vi "Calc Dev (DAQ Rack).vi"(0 "Verify Table IN":string[][](array[string]), 1 "Units":T2, 2 "Rack Version":T1, 5 "Dev Table 1 Ref":refnum<vi>) -> (14 "Verify Table OUT":string[][](array[string]))   [LabVIEW 2019]
uses:
  Type Defs/Units Type Def (DAQ Rack).ctl
  Type Defs/Rack Version Type Def.ctl
  <vilib>/Utility/miscctls.llb/LVRowAndColumnTypeDef.ctl
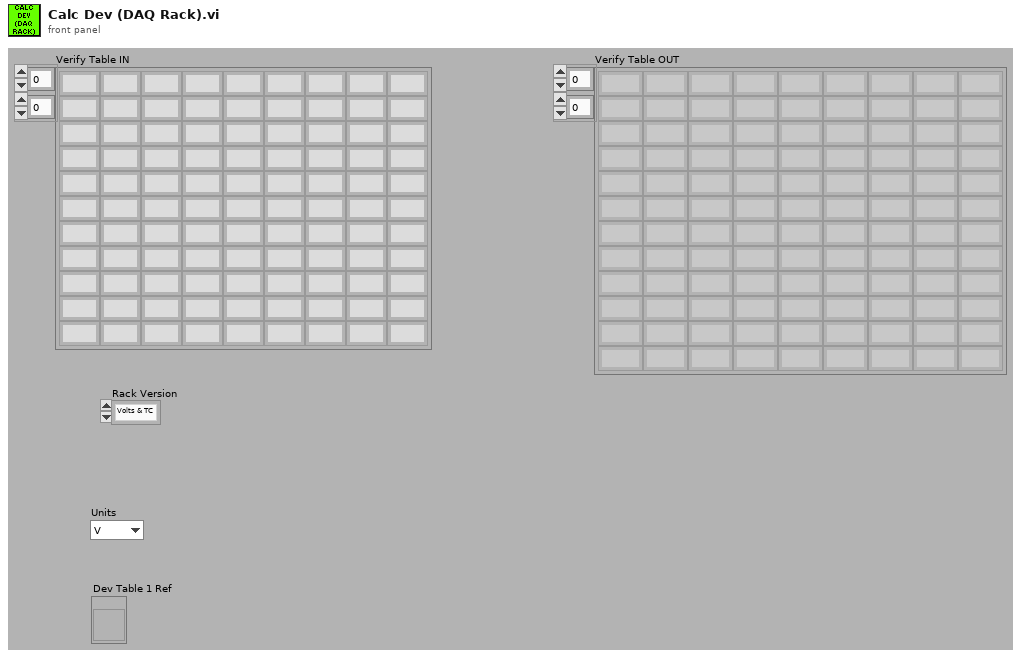
[diagram p1: front panel]
types:
  T1 = typedef "Rack Version Type Def.ctl" = enum16{"Volts & TC", "Volts", "RIO", "cDAQ", "Volts & Current", "Cart"}
  T2 = typedef "Units Type Def (DAQ Rack).ctl" = enum16{"V", "mA", "A", "Hz", "deg C"}
  T3 = typedef "LVRowAndColumnTypeDef.ctl" = cluster{"Row":i32, "Column":i32}
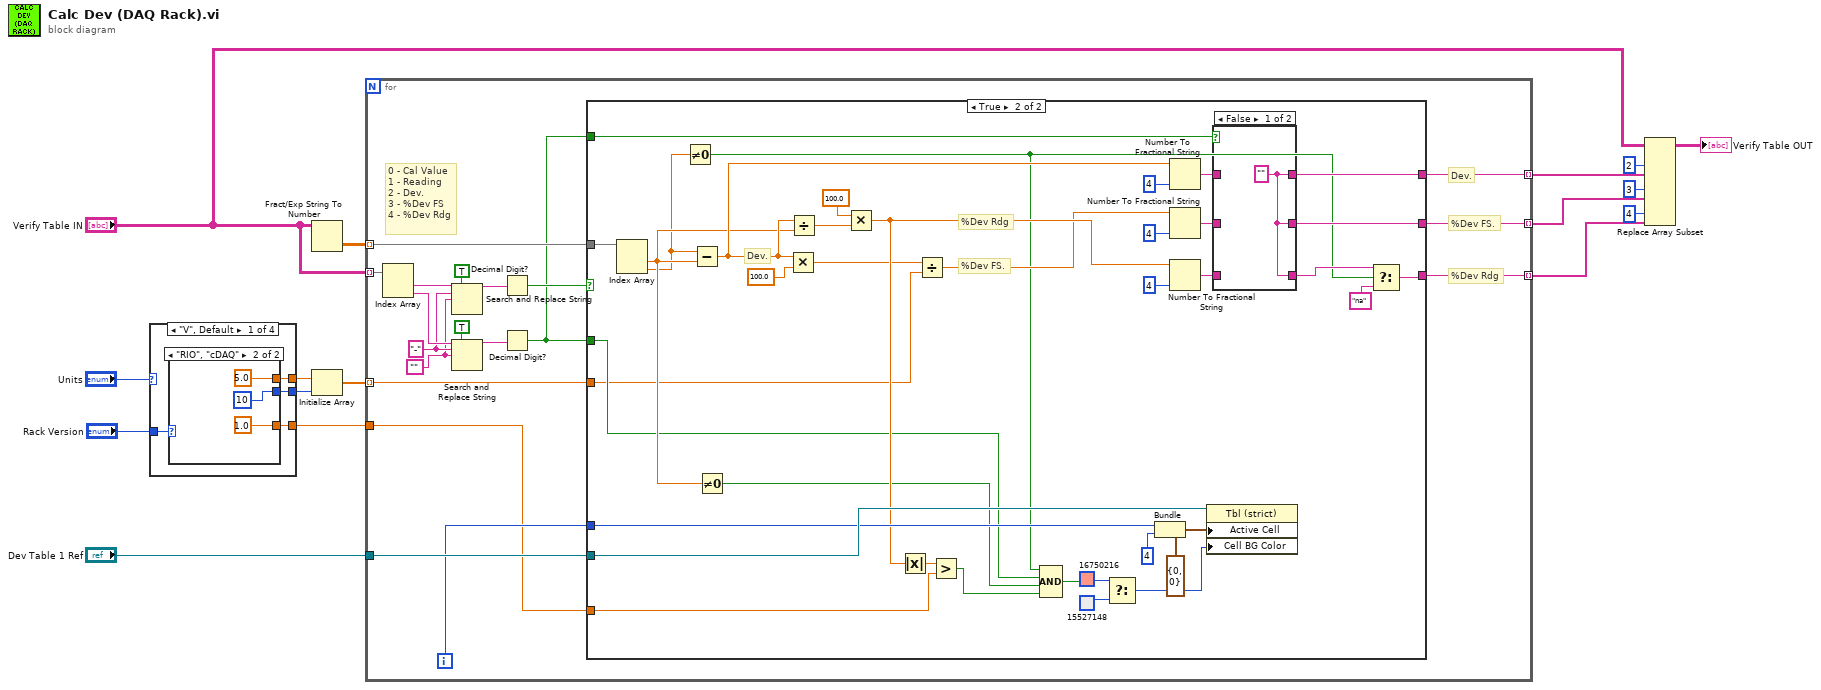
[diagram p0: block diagram]
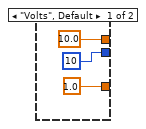
[diagram p2: hidden frame]
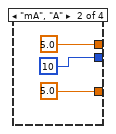
[diagram p3: hidden frame]
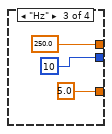
[diagram p4: hidden frame]
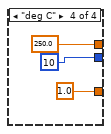
[diagram p5: hidden frame]
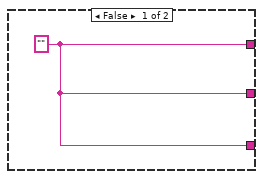
[diagram p6: hidden frame]
diagram:
  n1 = case shown="\"V\", Default" "Units" {
    tunnel: [w20 5.0 250.0 250.0] -> w14
    tunnel: [w19 10 ("dimension size") 10 ("dimension size") 10 ("dimension size")] -> w13
    tunnel: [w18 5.0 ("y") 5.0 ("y") 1.0 ("y")] -> w2
    tunnel: "Rack Version" -> [w17 _ _ _]
    frame "V", Default {
      n2 = case shown="\"RIO\", \"cDAQ\"" w17 {
        tunnel: [10.0 5.0] -> w20
        tunnel: [10 ("dimension size") 10 ("dimension size")] -> w19
        tunnel: [1.0 ("y") 1.0 ("y")] -> w18
        frame "Volts", Default {
        }
        frame "RIO", "cDAQ" {
        }
      }
    }
    frame "mA", "A" {
    }
    frame "Hz" {
    }
    frame "deg C" {
    }
  }
  n3 = Fract/Exp String To Number(string="Verify Table IN") -> (number=w16:dbl[][])  [unwired: 3 in, 1 out]
  n4 = Initialize Array(w14, w13) -> (w10:dbl[])
  n5 = for {
    tunnel: w16 -> [w53] mode=indexing
    tunnel: "Verify Table IN" -> [w54] mode=indexing
    tunnel: "Dev Table 1 Ref" -> [w52]
    tunnel: w10 -> [w48] mode=indexing
    tunnel: [w47] -> w7 mode=indexing
    tunnel: [w46] -> w6 mode=indexing
    tunnel: [w45] -> w5 mode=indexing
    tunnel: w2 -> [w36]
    i -> [w51]
    w37 = ""
    w38 = "-" ("search string")
    # "%Dev Rdg"
    # "%Dev FS."
    # "Dev."
    # "0 - Cal Value\n1 - Reading\n2 - Dev.\n3 - %Dev FS\n4 - %Dev Rdg"
    n6 = Index Array(array=w54) -> (element #1=w40:string, element #2=w44:string)  [unwired: 2 in]
    n7 = Search and Replace String(replace all?=TRUE ("replace all? (F)"), input string=w40, search string=w38, replace string=w37) -> (result string=w39:string)  [unwired: 4 in, 3 out]
    n8 = Search and Replace String(replace all?=TRUE ("replace all? (F)"), input string=w44, search string=w38, replace string=w37) -> (result string=w43:string)  [unwired: 4 in, 3 out]
    n9 = Decimal Digit?(1:w39) -> (0:w50:bool)
    n10 = Decimal Digit?(1:w43) -> (0:w49:bool)
    n11 = case shown="True" w50 {
      tunnel: w53 -> [_ w93]
      tunnel: [w55 w68] -> w47
      tunnel: [w55 w67] -> w46
      tunnel: [w55 w58] -> w45
      tunnel: w52 -> [_ w84]
      tunnel: w51 -> [_ w83]
      tunnel: w49 -> [_ w66]
      tunnel: w49 -> [_ w65]
      tunnel: w48 -> [_ w62]
      tunnel: w36 -> [_ w56]
      frame False {
        w55 = ""
      }
      frame True {
        # "%Dev Rdg"
        # "%Dev FS."
        # "Dev."
        n12 = Index Array(array=w93) -> (element #1=w73:dbl, element #2=w61:dbl)  [unwired: 2 in]
        n13 = Not Equal To 0?(x=w61) -> (x != 0?=w57:bool)
        n14 = Subtract(x=w61, y=w73) -> (x-y=w88:dbl)
        n15 = Not Equal To 0?(x=w73) -> (x != 0?=w72:bool)
        n16 = Multiply(x=w88, y=100.0) -> (x*y=w63:dbl)
        n17 = Divide(x=w88, y=w73) -> (x/y=w87:dbl)
        n18 = Multiply(x=100.0 ("y"), y=w87) -> (x*y=w76:dbl)
        n19 = Absolute Value(x=w76) -> (abs(x)=w85:dbl)
        n20 = Divide(x=w63, y=w62) -> (x/y=w64:dbl)
        n21 = Greater?(x=w85, y=w56) -> (0:w75:bool)
        n22 = Compound Arithmetic op=AND(w57, w65, w72, w75) -> (w74:bool)
        n23 = Select(t=u32 16750216, s=w74, f=u32 15527148) -> (s? t:f=w77:u32)
        n24 = Bundle(cluster=T3 {"Row"=0, "Column"=0} ("Active Cell:Active Cell"), "Row"=w83, "Column"=4) -> (w81:T3)
        n25 = Number To Fractional String(number=w88, precision (6)=i16 4) -> (F-format string=w71:string)  [unwired: 2 in]
        n26 = Number To Fractional String(number=w64, precision (6)=i16 4) -> (F-format string=w70:string)  [unwired: 2 in]
        n27 = Number To Fractional String(number=w76, precision (6)=i16 4) -> (F-format string=w69:string)  [unwired: 2 in]
        n28 = property on="Property Node" class="Tbl (strict)"(reference=w84, "Active Cell"=w81, "Cell BG Color"=w77) -> ()  [unwired: 1 in, 2 out]
        n29 = case shown="False" w66 {
          tunnel: [w94 w97] -> w68
          tunnel: w71 -> [_ w97]
          tunnel: w70 -> [_ w96]
          tunnel: [w94 w96] -> w67
          tunnel: w69 -> [_ w95]
          tunnel: [w94 w95] -> w59
          frame False {
            w94 = ""
          }
          frame True {
          }
        }
        n30 = Select(t=w59, s=w57, f="na") -> (s? t:f=w58:string)
      }
    }
  }
  n31 = Replace Array Subset(array="Verify Table IN", new element #1=w7, index (col) #1=2 ("disabled index (col)"), new element #2=w6, index (col) #2=3 ("disabled index (col)"), new element #3=w5, index (col) #3=4 ("disabled index (col)")) -> (→"Verify Table OUT":string[][])  [unwired: 3 in]
